vi "tm3samp_08a_dcimgtotiff_wVision.vi"() -> ()   [LabVIEW 2023]
panel:
  out "Error Out":errorcluster
  out "Files written to":path
  out "Index":i32
  out "Total":i32
  in  "DCIMG Path":path
  # "This is an example of how to read the images\nwithin a DCIMG file and write them to TIFF files."
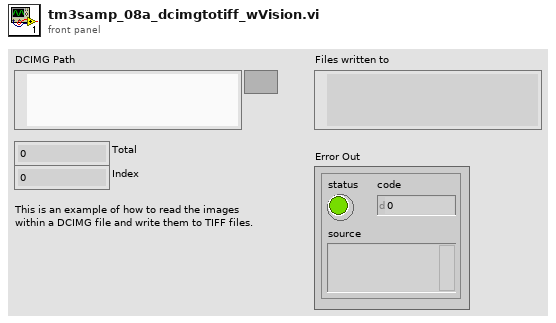
[diagram p1: front panel]
types:
  T1 = typedef "Image Type" = u32
  T2 = typedef "IMAQ Image.ctl" = refnum<image>
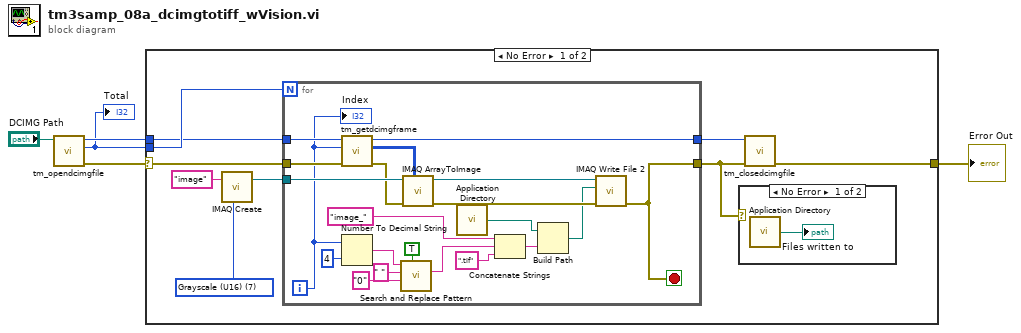
[diagram p0: block diagram]
diagram:
  n1 = call "tm_opendcimgfile.vi"("Path"="DCIMG Path") -> ("error out"=w5:errorcluster, "Total Frames"=w2:i32, "File Handle"=w4:u32)  [unwired: 8 in]
  "Total" <- w2
  n2 = case shown="No Error" w5 {
    selector: w5 -> [w11 w37]
    tunnel: w4 -> [w12 _]
    tunnel: [w14 w37] -> w1
    tunnel: w2 -> [w13 _]
    frame No Error {
      w9 = T1 7 items=["Grayscale (U8)", "Grayscale (I16)", "Grayscale (SGL)", "Complex (CSG)", "RGB (U32)", "HSL (U32)", "RGB (U64)", "Grayscale (U16)"] ("Image Type")
      n3 = call "IMAQ Create"("Image Name"="image", "Image Type"=w9) -> ("New Image"=w8:T2)  [unwired: 3 in, 1 out]
      n4 = for {
        N: w13 -> [_]
        tunnel: w12 -> [w36]
        tunnel: w11 -> [w35]
        tunnel: w8 -> [w34]
        tunnel: [w16] -> w6
        tunnel: [w30] -> w7
        i -> [w17]
        stop <- w16 stop-if-true
        n5 = call "tm_getdcimgframe.vi"("error in (no error)"=w35, "Frame Index"=w17, "File Handle in"=w36) -> ("error out"=w31:errorcluster, "Data"=w18:u16[][], "File Handle out"=w30:u32)  [unwired: 5 in, 1 out]
        n6 = Number To Decimal String(number=w17, width (-)=i16 4) -> (decimal integer string=w27:string)
        n7 = call <vilib>:"Search and Replace Pattern.vi"("string"=w27, "regular expression (\"\")"=" " ("regular expression (\"\")"), "replace string (\"\")"="0" ("replace string (\"\")"), "replace all? (F)"=TRUE) -> ("result string"=w23:string)  [unwired: 1 in, 1 out]
        n8 = call "IMAQ ArrayToImage"("Image Pixels (U16)"=w18, "error in (no error)"=w31, "Image"=w34) -> ("error out"=w33:errorcluster, "Image Out"=w32:T2)  [unwired: 7 in]
        n9 = call <vilib>:"Application Directory.vi"() -> ("Application Directory"=w19:path)
        n10 = Concatenate Strings("image_", w23, ".tif" ("regular expression (\"\")")) -> (w22:string)
        n11 = Build Path(base path=w19, name or relative path=w22) -> (appended path=w21:path)
        n12 = call-poly "IMAQ Write File 2"("error in (no error)"=w33, "File Path"=w21, "Image"=w32) -> ("error out"=w16:errorcluster)  [unwired: 7 in, 1 out]
        "Index" <- w17
      }
      n13 = case shown="No Error" w6 {
        frame No Error {
          n14 = call <vilib>:"Application Directory.vi"() -> ("Application Directory"=→"Files written to":path)
        }
        frame Error {
        }
      }
      n15 = call "tm_closedcimgfile.vi"("error in (no error)"=w6, "File Handle"=w7) -> ("error out"=w14:errorcluster)  [unwired: 9 in]
    }
    frame Error {
    }
  }
  "Error Out" <- w1
